vi "readForm.vi"(1 "httpRequestID":u32) -> (0 "output cluster":T1)   [LabVIEW 2011]
uses:
  <vilib>/wsapi/NI_WebServices.lvlib
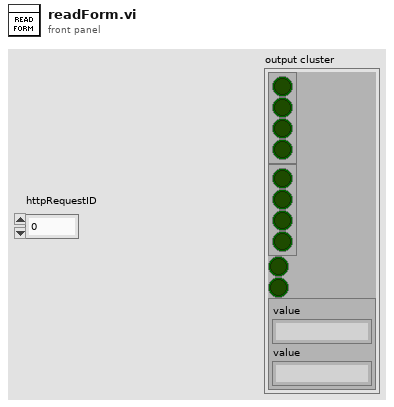
[diagram p1: front panel]
types:
  T1 = cluster{cluster{bool, bool, bool, bool}, cluster{bool, bool, bool, bool}, bool, bool, cluster{"value":string, "value":string}}
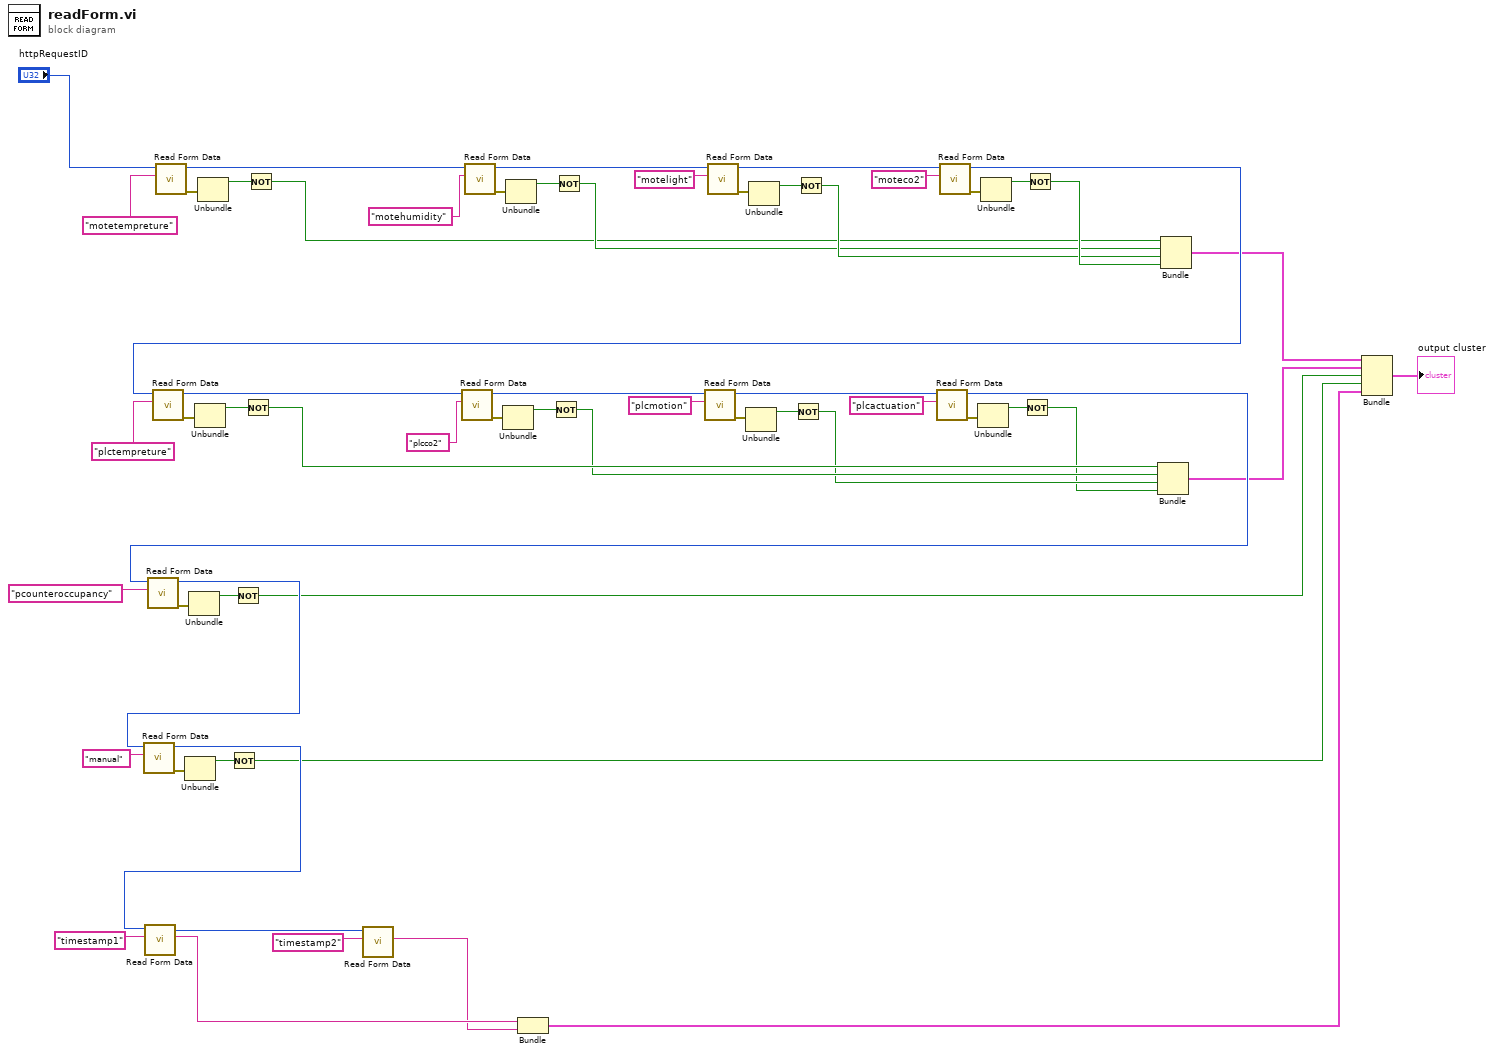
[diagram p0: block diagram]
diagram:
  n1 = call <vilib>:"Read Form Data.vi"("key"="motetempreture", "httpRequestID"="httpRequestID") -> ("error out"=w24:errorcluster, "httpRequestID out"=w21:u32)  [unwired: 1 in, 7 out]
  n2 = Unbundle(w24) -> ("status"=w28:bool)  [unwired: 2 out]
  n3 = Not(x=w28) -> (.not. x?=w32:bool)
  n4 = call <vilib>:"Read Form Data.vi"("key"="motehumidity", "httpRequestID"=w21) -> ("error out"=w25:errorcluster, "httpRequestID out"=w22:u32)  [unwired: 1 in, 7 out]
  n5 = Unbundle(w25) -> ("status"=w29:bool)  [unwired: 2 out]
  n6 = Not(x=w29) -> (.not. x?=w33:bool)
  n7 = call <vilib>:"Read Form Data.vi"("key"="motelight", "httpRequestID"=w22) -> ("error out"=w26:errorcluster, "httpRequestID out"=w23:u32)  [unwired: 1 in, 7 out]
  n8 = Unbundle(w26) -> ("status"=w30:bool)  [unwired: 2 out]
  n9 = Not(x=w30) -> (.not. x?=w34:bool)
  n10 = call <vilib>:"Read Form Data.vi"("key"="moteco2", "httpRequestID"=w23) -> ("error out"=w27:errorcluster, "httpRequestID out"=w12:u32)  [unwired: 1 in, 7 out]
  n11 = call <vilib>:"Read Form Data.vi"("key"="plctempreture", "httpRequestID"=w12) -> ("error out"=w53:errorcluster, "httpRequestID out"=w56:u32)  [unwired: 1 in, 7 out]
  n12 = Unbundle(w53) -> ("status"=w49:bool)  [unwired: 2 out]
  n13 = Not(x=w49) -> (.not. x?=w45:bool)
  n14 = call <vilib>:"Read Form Data.vi"("key"="plcco2", "httpRequestID"=w56) -> ("error out"=w52:errorcluster, "httpRequestID out"=w55:u32)  [unwired: 1 in, 7 out]
  n15 = Unbundle(w52) -> ("status"=w48:bool)  [unwired: 2 out]
  n16 = Not(x=w48) -> (.not. x?=w44:bool)
  n17 = call <vilib>:"Read Form Data.vi"("key"="plcmotion", "httpRequestID"=w55) -> ("error out"=w51:errorcluster, "httpRequestID out"=w54:u32)  [unwired: 1 in, 7 out]
  n18 = Unbundle(w51) -> ("status"=w47:bool)  [unwired: 2 out]
  n19 = Not(x=w47) -> (.not. x?=w43:bool)
  n20 = call <vilib>:"Read Form Data.vi"("key"="plcactuation", "httpRequestID"=w54) -> ("error out"=w50:errorcluster, "httpRequestID out"=w11:u32)  [unwired: 1 in, 7 out]
  n21 = call <vilib>:"Read Form Data.vi"("key"="pcounteroccupancy", "httpRequestID"=w11) -> ("error out"=w37:errorcluster, "httpRequestID out"=w10:u32)  [unwired: 1 in, 7 out]
  n22 = call <vilib>:"Read Form Data.vi"("key"="manual", "httpRequestID"=w10) -> ("error out"=w14:errorcluster, "httpRequestID out"=w9:u32)  [unwired: 1 in, 7 out]
  n23 = call <vilib>:"Read Form Data.vi"("key"="timestamp1", "httpRequestID"=w9) -> ("value"=w2:string, "httpRequestID out"=w39:u32)  [unwired: 1 in, 7 out]
  n24 = Unbundle(w14) -> ("status"=w13:bool)  [unwired: 2 out]
  n25 = Unbundle(w37) -> ("status"=w38:bool)  [unwired: 2 out]
  n26 = Not(x=w13) -> (.not. x?=w5:bool)
  n27 = Not(x=w38) -> (.not. x?=w6:bool)
  n28 = call <vilib>:"Read Form Data.vi"("key"="timestamp2", "httpRequestID"=w39) -> ("value"=w1:string)  [unwired: 1 in, 8 out]
  n29 = Bundle("value"=w2, "value"=w1) -> (w4:cluster{"value":string, "value":string})  [unwired: 1 in]
  n30 = Unbundle(w50) -> ("status"=w46:bool)  [unwired: 2 out]
  n31 = Unbundle(w27) -> ("status"=w31:bool)  [unwired: 2 out]
  n32 = Not(x=w46) -> (.not. x?=w42:bool)
  n33 = Not(x=w31) -> (.not. x?=w35:bool)
  n34 = Bundle(w45, w44, w43, w42) -> (w7:cluster{bool, bool, bool, bool})  [unwired: 1 in]
  n35 = Bundle(w32, w33, w34, w35) -> (w8:cluster{bool, bool, bool, bool})  [unwired: 1 in]
  n36 = Bundle(w8, w7, w6, w5, w4) -> (→"output cluster":T1)  [unwired: 1 in]
